vi "Translate to Array Data_BU2.vi"(8 "modified error":errorcluster, 9 "modified data":path=path "C:/Users/User/Desktop/test.csv", 10 "original error":errorcluster, 11 "original data":path=path "C:/Users/User/Desktop/aaa.csv") -> ()   [LabVIEW 2023]
uses:
  <vilib>/Utility/error.llb/DialogType.ctl
panel:
  in  "Electrode number, N":u16=8
  out "number 2":i32
  out "number":i32
  in  "Only Use Last Value?":bool=TRUE
  in  "Array Mode":u16(ring) items=["Gradient + Dipole dipole", "Gradient", "Dipole Dipole", "Schlumberger"]
  in  "Insert\nBreak":bool=TRUE
  in  "Inverse\nPolarity":bool=TRUE
  in  "Current Mode":u8[][](array[numeric])
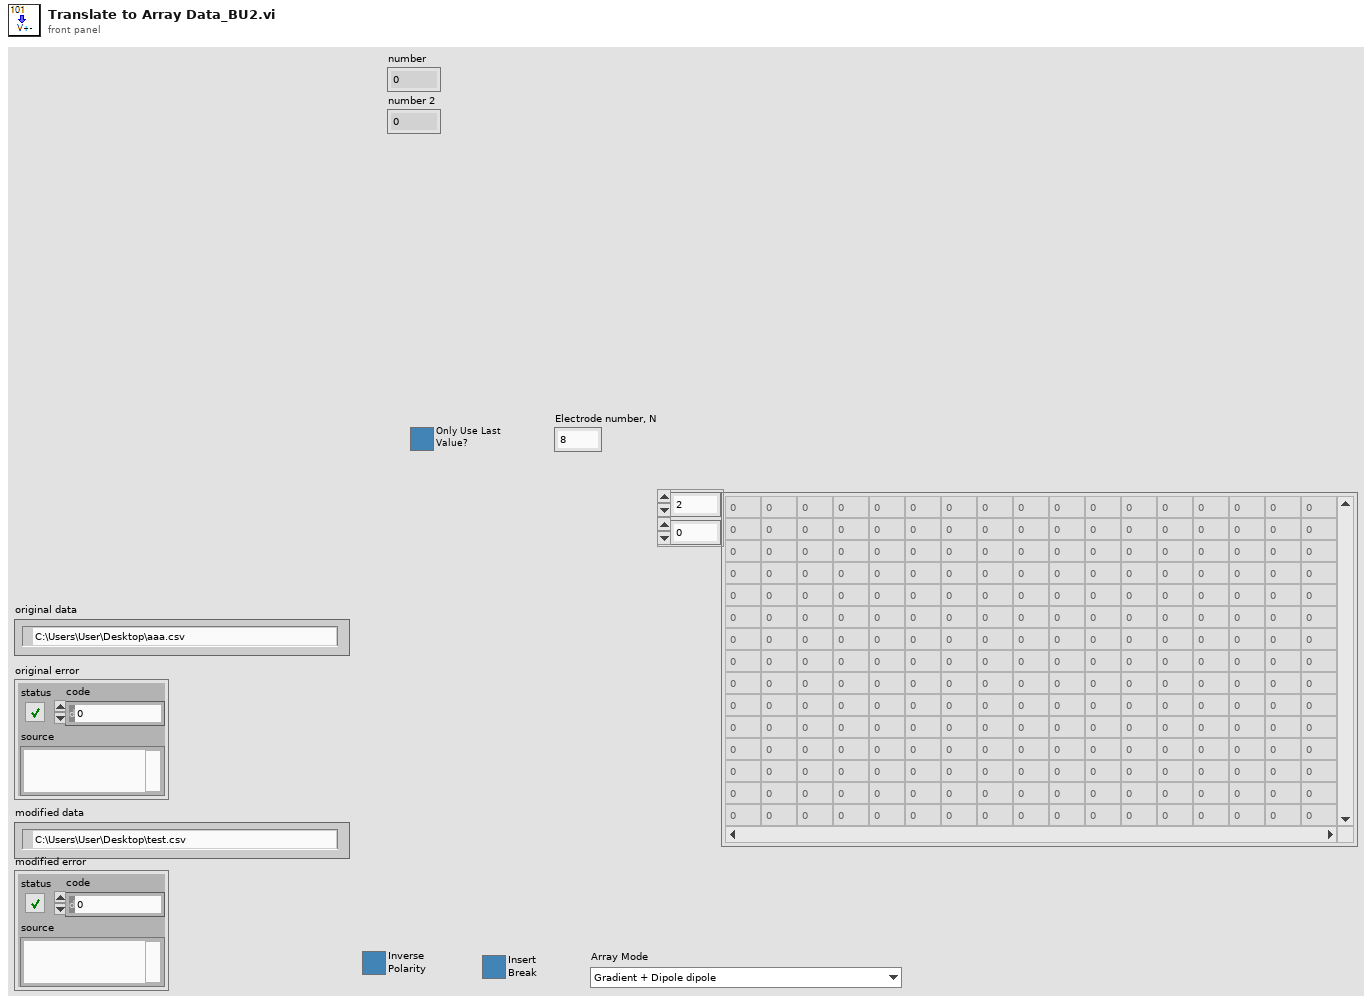
[diagram p1: front panel]
types:
  T1 = enum16{"open", "replace", "create", "open or create", "replace or create", "replace or create with confirmation"}
  T2 = typedef "DialogType.ctl" = u16
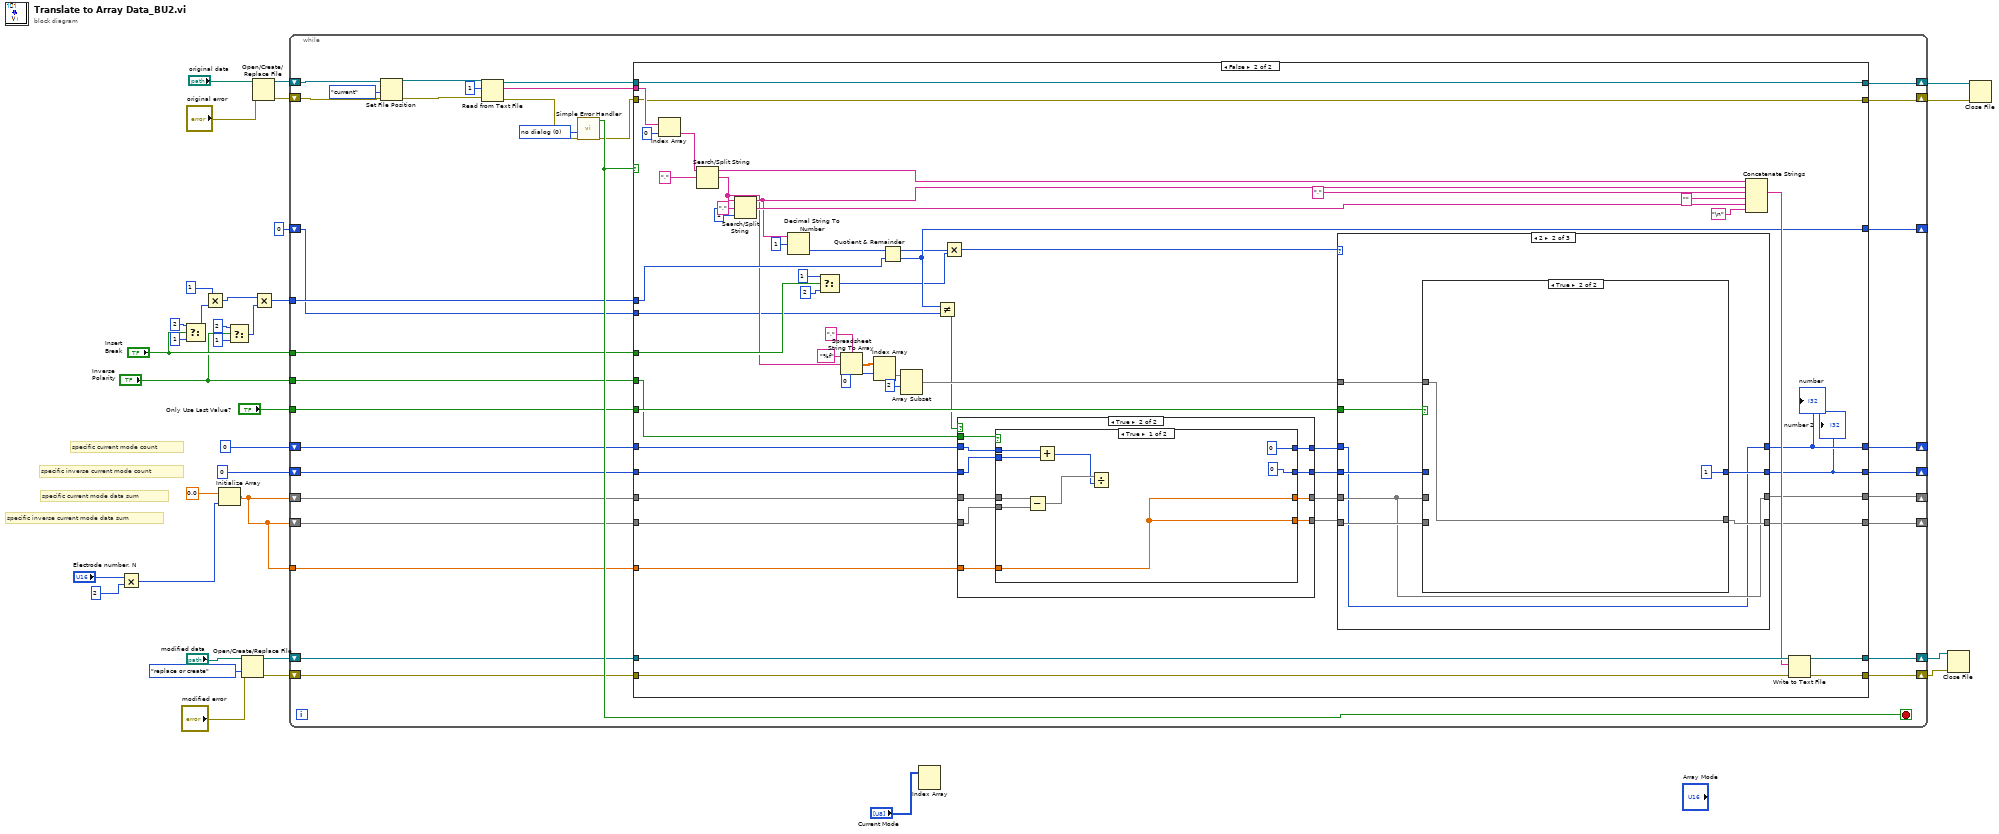
[diagram p0: block diagram]
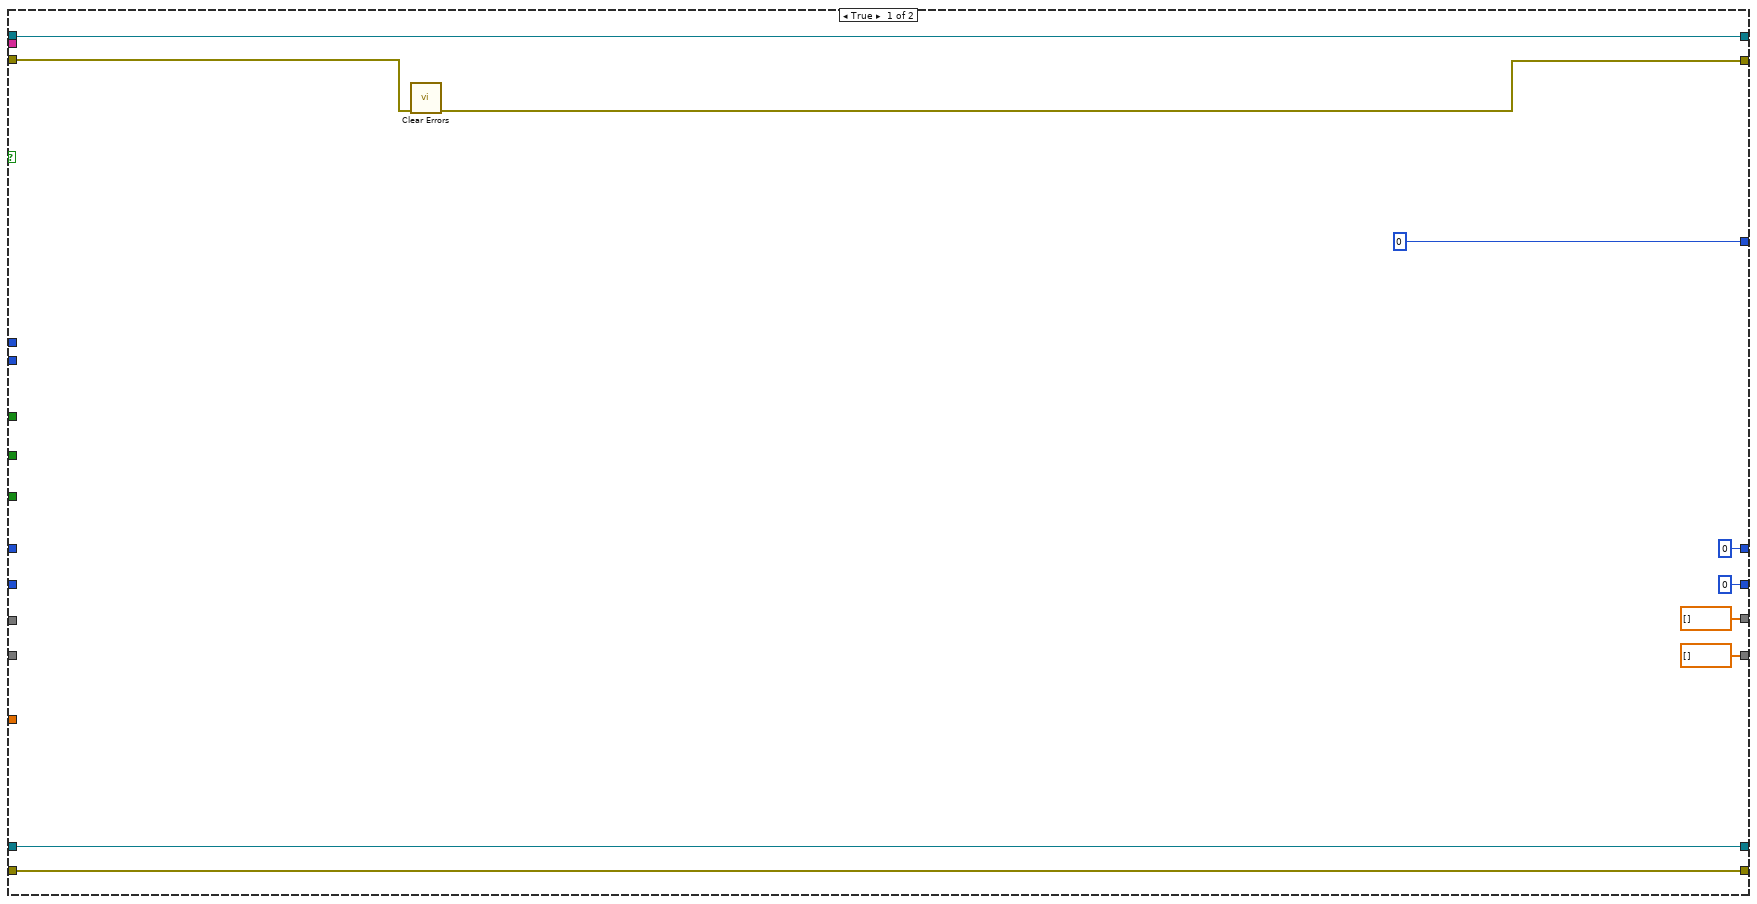
[diagram p2: hidden frame]
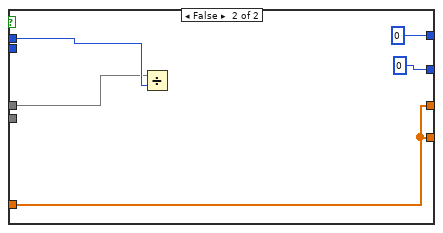
[diagram p4: hidden frame]
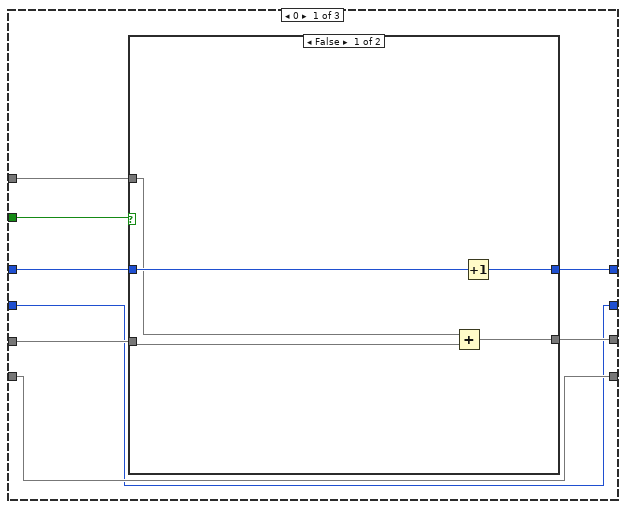
[diagram p5: hidden frame]
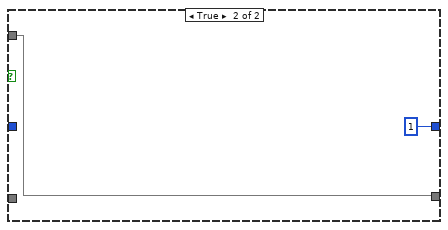
[diagram p6: hidden frame]
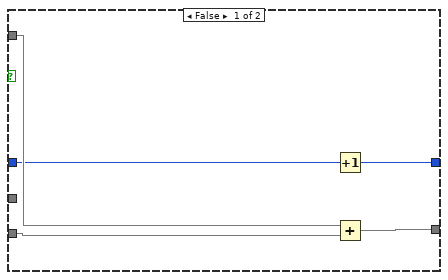
[diagram p7: hidden frame]
diagram:
  # "specific inverse current mode data sum"
  # "specific current mode data sum"
  # "specific inverse current mode count"
  # "specific current mode count"
  n1 = Multiply(x="Electrode number, N", y=u16 2) -> (x*y=w2:u16)
  n2 = Select(t=2 ("number"), s="Insert\nBreak", f=1 ("number")) -> (s? t:f=w12:i32)
  n3 = Multiply(x=1 ("number"), y=w12) -> (x*y=w6:i32)
  n4 = Initialize Array(0.0 ("element"), w2) -> (w1:dbl[])
  n5 = Select(t=2 ("number"), s="Inverse\nPolarity", f=1 ("number")) -> (s? t:f=w11:i32)
  n6 = Open/Create/Replace File(file path (use dialog)="modified data", error in="modified error", operation (0:open)=T1."replace or create") -> (refnum out=w29:refnum<file>, error out=w28:errorcluster)  [unwired: 3 in, 1 out]
  n7 = Open/Create/Replace File(file path (use dialog)="original data", error in="original error") -> (refnum out=w31:refnum<file>, error out=w32:errorcluster)  [unwired: 4 in, 1 out]
  n8 = Multiply(x=w6, y=w11) -> (x*y=w10:i32)
  n9 = while {
    shift-right: [w59] -> w22
    shift-left: w32 -> [w66]
    shift-right: [w58] -> w33
    shift-left: w31 -> [w57]
    shift-right: [w52] -> w24
    shift-left: w29 -> [w54]
    shift-right: [w51] -> w23
    shift-left: w28 -> [w53]
    tunnel: "Insert\nBreak" -> [w49]
    tunnel: "Inverse\nPolarity" -> [w48]
    tunnel: "Only Use Last Value?" -> [w47]
    tunnel: w10 -> [w46]
    shift-right: [w41] -> _
    shift-left: 0 ("number") -> [w45]
    shift-right: [w38] -> _
    shift-left: 0 ("number") -> [w44]
    shift-right: [w40] -> _
    shift-left: w1 -> [w43]
    shift-right: [w39] -> _
    shift-left: w1 -> [w42]
    shift-right: [w37] -> _
    shift-left: 0 -> [w36]
    tunnel: w1 -> [w35]
    stop <- w63 stop-if-true
    w64 = T2 0 items=["no dialog", "OK message", "continue or stop message", "OK message + warnings", "continue/stop + warnings"] ("type of dialog (OK msg:1)")
    n10 = Set File Position(refnum=w57, from (0:start)=enum16{"start", "end", "current"}."current", error in=w66) -> (refnum out=w56:refnum<file>, error out=w55:errorcluster)  [unwired: 1 in]
    n11 = Read from Text File(file (use dialog)=w56, count=1, error in=w55) -> (refnum out=w61:refnum<file>, text=w62:string[], error out=w60:errorcluster)  [unwired: 1 in, 1 out]
    n12 = call <vilib>:"Simple Error Handler.vi"("type of dialog (OK msg:1)"=w64, "error in (no error)"=w60) -> ("error?"=w63:bool, "error out"=w50:errorcluster)  [unwired: 3 in, 3 out]
    n13 = case shown="False" w63 {
      tunnel: w62 -> [_ w125]
      tunnel: w61 -> [w77 w122]
      tunnel: w50 -> [w74 w121]
      tunnel: [w77 w122] -> w58
      tunnel: [w73 w121] -> w59
      tunnel: w54 -> [w76 w120]
      tunnel: w53 -> [w75 w119]
      tunnel: [w76 w118] -> w52
      tunnel: [w75 w117] -> w51
      tunnel: w49 -> [_ w111]
      tunnel: w48 -> [_ w88]
      tunnel: w47 -> [_ w108]
      tunnel: w46 -> [_ w109]
      tunnel: w45 -> [_ w92]
      tunnel: w44 -> [_ w91]
      tunnel: w43 -> [_ w90]
      tunnel: w42 -> [_ w89]
      tunnel: [0 ("number") w98] -> w41
      tunnel: [dbl[] [] ("subarray") w97] -> w40
      tunnel: [dbl[] [] ("subarray") w96] -> w39
      tunnel: [0 ("number") w95] -> w38
      tunnel: [0 w93] -> w37
      tunnel: w36 -> [_ w94]
      tunnel: w35 -> [_ w82]
      frame True {
        n14 = call <vilib>:"Clear Errors.vi"("error in (no error)"=w74) -> ("error out"=w73:errorcluster)  [unwired: 5 in, 1 out]
      }
      frame False {
        n15 = Index Array(array=w125, index=0) -> (element=w123:string)
        n16 = Search/Split String(string=w123, search string/char (-)=",") -> (substring before match=w131:string, match + rest of string=w104:string)  [unwired: 1 in, 1 out]
        n17 = Search/Split String(string=w104, search string/char (-)=",", offset (0)=1) -> (substring before match=w105:string, match + rest of string=w114:string)  [unwired: 1 out]
        n18 = Decimal String To Number(string=w105, offset=1) -> (number=w81:i32)  [unwired: 1 in, 1 out]
        n19 = Select(t=1, s=w111, f=2 ("y")) -> (s? t:f=w80:i32)
        n20 = Spreadsheet String To Array(delimiter (Tab)=",", format string="%f", spreadsheet string=w104) -> (array=w103:dbl[][])  [unwired: 1 in]
        n21 = Index Array(array=w103, index (row)=0) -> (element=w101:dbl[])  [unwired: 1 in]
        n22 = Quotient & Remainder(x=w81, y=w109) -> (x-y*floor(x/y)=w79:i32, floor(x/y)=w93:i32)
        n23 = Array Subset(array=w101, index=2) -> (w99:dbl[])  [unwired: 1 in]
        n24 = Not Equal?(x=w93, y=w94) -> (x != y?=w83:bool)
        n25 = Multiply(x=w79, y=w80) -> (x*y=w78:i32)
        n26 = case shown="True" w83 {
          tunnel: w92 -> [w135 w142]
          tunnel: w91 -> [w134 w141]
          tunnel: w90 -> [w133 w144]
          tunnel: w89 -> [w132 w143]
          tunnel: w88 -> [_ w145]
          tunnel: [w135 w140] -> w87
          tunnel: [w134 w139] -> w86
          tunnel: [w133 w138] -> w85
          tunnel: [w132 w137] -> w84
          tunnel: w82 -> [_ w136]
          frame False {
          }
          frame True {
            n27 = case shown="True" w145 {
              tunnel: w144 -> [w154 w156]
              tunnel: w143 -> [w153 _]
              tunnel: w142 -> [w152 w157]
              tunnel: w141 -> [w151 _]
              tunnel: [0 ("number") 0 ("number")] -> w140
              tunnel: [0 ("number") 0 ("number")] -> w139
              tunnel: [w146 w155] -> w138
              tunnel: [w146 w155] -> w137
              tunnel: w136 -> [w146 w155]
              frame True {
                n28 = Subtract(x=w154, y=w153) -> (x-y=w150:dbl[])
                n29 = Add(x=w152, y=w151) -> (x+y=w149:i32)
                n30 = Divide(x=w150, y=w149) -> ()  [unwired: 1 out]
              }
              frame False {
                n31 = Divide(x=w156, y=w157) -> ()  [unwired: 1 out]
              }
            }
          }
        }
        n32 = case shown="2" w78 {
          tunnel: w108 -> [w167 w182 _]
          tunnel: w99 -> [w163 w181 _]
          tunnel: w87 -> [w166 w175 w193]
          tunnel: w86 -> [w160 w178 w192]
          tunnel: w85 -> [w165 w176 w191]
          tunnel: w84 -> [w161 w180 w190]
          tunnel: [w164 w175 w193] -> w98
          tunnel: [w162 w176 w191] -> w97
          tunnel: [w161 w179 w190] -> w96
          tunnel: [w160 w177 w192] -> w95
          frame 0 {
            n33 = case shown="False" w167 {
              tunnel: w166 -> [w172 _]
              tunnel: w165 -> [w169 _]
              tunnel: [w171 1 ("number")] -> w164
              tunnel: w163 -> [w168 w173]
              tunnel: [w170 w173] -> w162
              frame False {
                n34 = Add(x=w168, y=w169) -> (x+y=w170:dbl[])
                n35 = Increment(x=w172) -> (x+1=w171:i32)
              }
              frame True {
              }
            }
          }
          frame 2 {
            n36 = case shown="True" w182 {
              tunnel: w176 -> [_ _]
              tunnel: w181 -> [w186 w189]
              tunnel: [w187 w189] -> w179
              tunnel: w180 -> [w185 _]
              tunnel: w178 -> [w184 _]
              tunnel: [w183 1 ("number")] -> w177
              frame False {
                n37 = Increment(x=w184) -> (x+1=w183:i32)
                n38 = Add(x=w186, y=w185) -> (x+y=w187:dbl[])
              }
              frame True {
              }
            }
          }
          frame 1, 3, Default {
          }
        }
        "number" <- w98
        "number 2" <- w95
        n39 = Concatenate Strings(w131, w105, "," ("string"), "" ("string"), w114, "\n") -> (w116:string)
        n40 = Write to Text File(file (use dialog)=w120, text=w116, error in=w119) -> (refnum out=w118:refnum<file>, error out=w117:errorcluster)  [unwired: 1 in, 1 out]
      }
    }
  }
  n41 = Index Array(array="Current Mode") -> ()  [unwired: 2 in, 1 out]
  n42 = Close File(refnum=w24, error in=w23) -> ()  [unwired: 2 out]
  n43 = Close File(refnum=w33, error in=w22) -> ()  [unwired: 2 out]
